vi "FindClassNamesParentAndStart.vi"(8 "error in (no error)":errorcluster, 10 "baseClass":refnum<class "baseClass.lvclass">, 11 "CS in":refnum<class "CS.lvclass">) -> (0 "error out":errorcluster, 3 "CS out":refnum<class "CS.lvclass">)   [LabVIEW 2013, in "CS.lvclass"]
uses:
  CS.lvclass
  baseClass/baseClass.lvclass
  <vilib>/Utility/error.llb/whitespace.ctl
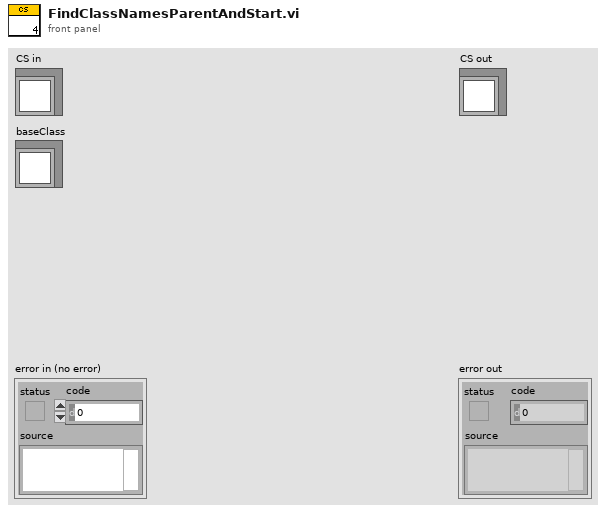
[diagram p1: front panel]
types:
  T1 = typedef "whitespace.ctl" = u16
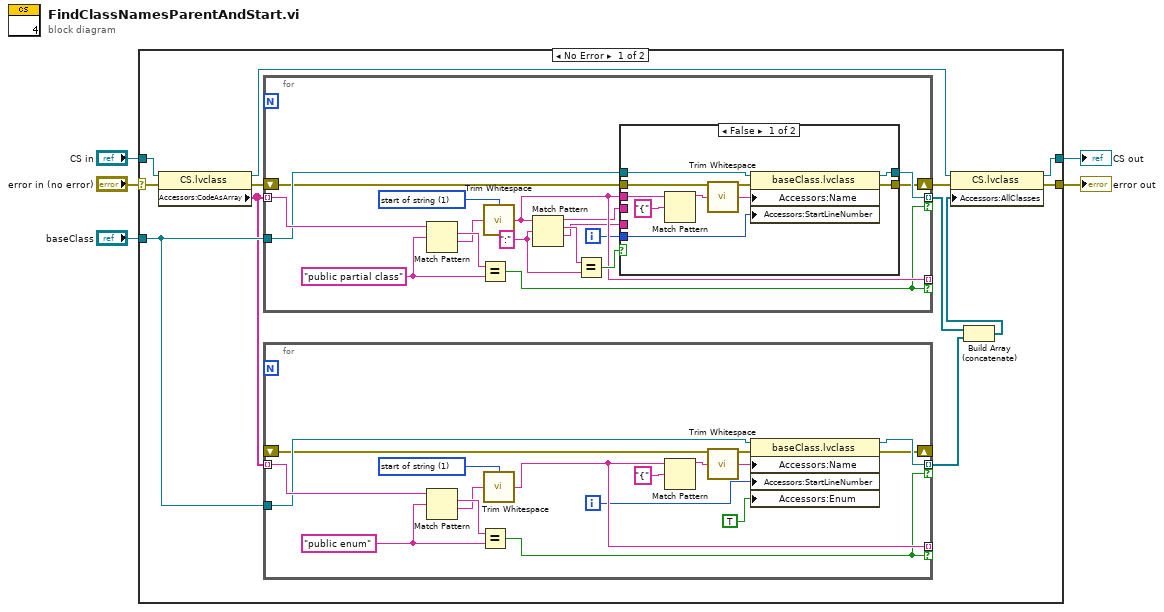
[diagram p0: block diagram]
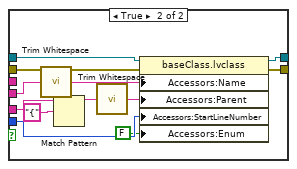
[diagram p2: hidden frame]
diagram:
  n1 = case shown="No Error" "error in (no error)" {
    selector: "error in (no error)" -> [w14 w73]
    tunnel: [w11 w73] -> w4
    tunnel: [w13 w72] -> w2
    tunnel: "CS in" -> [w17 w72]
    tunnel: "baseClass" -> [w10 _]
    frame No Error {
      n2 = property class="CS.lvclass"(reference=w17, error in=w14) -> (reference out=w16:refnum<class "CS.lvclass">, error out=w15:errorcluster, "Accessors:CodeAsArray"=w9:string[])
      n3 = for {
        tunnel: w9 -> [w50] mode=indexing
        tunnel: [w41] -> _ mode=indexing if=w37
        tunnel: w10 -> [w42]
        tunnel: [w38] -> w8 mode=indexing if=w37
        shift-right: [w34] -> w12
        shift-left: w15 -> [w35]
        i -> [w36]
        w44 = ":" ("regular expression")
        w47 = T1 1 items=["both", "start of string", "end of string"] ("location (both)")
        w48 = "public partial class"
        n4 = Match Pattern(string=w50, regular expression=w48) -> (match substring=w49:string, after substring=w46:string)  [unwired: 1 in, 2 out]
        n5 = Equal?(x=w49, y=w48) -> (x = y?=w37:bool)
        n6 = call <vilib>:"Trim Whitespace.vi"("string"=w46, "location (both)"=w47) -> ("trimmed string"=w41:string)
        n7 = Match Pattern(string=w41, regular expression=w44) -> (before substring=w40:string, match substring=w45:string, after substring=w39:string)  [unwired: 1 in, 1 out]
        n8 = Equal?(x=w45, y=w44) -> (x = y?=w43:bool)
        n9 = case shown="False" w43 {
          tunnel: w42 -> [w59 w71]
          tunnel: w41 -> [w58 _]
          tunnel: w40 -> [_ w70]
          tunnel: w39 -> [_ w69]
          tunnel: [w55 w66] -> w38
          tunnel: w36 -> [w53 w63]
          tunnel: w35 -> [w51 w62]
          tunnel: [w52 w61] -> w34
          frame False {
            n10 = Match Pattern(string=w58, regular expression="{") -> (before substring=w56:string)  [unwired: 1 in, 3 out]
            n11 = call <vilib>:"Trim Whitespace.vi"("string"=w56) -> ("trimmed string"=w54:string)  [unwired: 1 in]
            n12 = property class="baseClass.lvclass"(reference=w59, error in=w51, "Accessors:Name"=w54, "Accessors:StartLineNumber"=w53) -> (reference out=w55:refnum<class "baseClass.lvclass">, error out=w52:errorcluster)
          }
          frame True {
            n13 = call <vilib>:"Trim Whitespace.vi"("string"=w70) -> ("trimmed string"=w64:string)  [unwired: 1 in]
            n14 = Match Pattern(string=w69, regular expression="{") -> (before substring=w67:string)  [unwired: 1 in, 3 out]
            n15 = call <vilib>:"Trim Whitespace.vi"("string"=w67) -> ("trimmed string"=w65:string)  [unwired: 1 in]
            n16 = property class="baseClass.lvclass"(reference=w71, error in=w62, "Accessors:Name"=w64, "Accessors:Parent"=w65, "Accessors:StartLineNumber"=w63, "Accessors:Enum"=FALSE ("Enum")) -> (reference out=w66:refnum<class "baseClass.lvclass">, error out=w61:errorcluster)
          }
        }
      }
      n17 = for {
        tunnel: w9 -> [w33] mode=indexing
        tunnel: [w27] -> _ mode=indexing if=w25
        tunnel: w10 -> [w28]
        tunnel: [w26] -> w7 mode=indexing if=w25
        shift-right: [w22] -> _
        shift-left: _ -> [w23]
        i -> [w24]
        w30 = T1 1 items=["both", "start of string", "end of string"] ("location (both)")
        w31 = "public enum"
        n18 = Match Pattern(string=w33, regular expression=w31) -> (match substring=w32:string, after substring=w29:string)  [unwired: 1 in, 2 out]
        n19 = Equal?(x=w32, y=w31) -> (x = y?=w25:bool)
        n20 = call <vilib>:"Trim Whitespace.vi"("string"=w29, "location (both)"=w30) -> ("trimmed string"=w27:string)
        n21 = Match Pattern(string=w27, regular expression="{") -> (before substring=w20:string)  [unwired: 1 in, 3 out]
        n22 = call <vilib>:"Trim Whitespace.vi"("string"=w20) -> ("trimmed string"=w19:string)  [unwired: 1 in]
        n23 = property class="baseClass.lvclass"(reference=w28, error in=w23, "Accessors:Name"=w19, "Accessors:StartLineNumber"=w24, "Accessors:Enum"=TRUE ("Enum")) -> (reference out=w26:refnum<class "baseClass.lvclass">, error out=w22:errorcluster)
      }
      n24 = Build Array (concatenate)(w8, w7) -> (w6:refnum<class "baseClass.lvclass">[])
      n25 = property class="CS.lvclass"(reference=w16, error in=w12, "Accessors:AllClasses"=w6) -> (reference out=w13:refnum<class "CS.lvclass">, error out=w11:errorcluster)
    }
    frame Error {
    }
  }
  "error out" <- w4
  "CS out" <- w2
